vi "Write Kill Methods On Exit.vi"(8 "error in (no error)":errorcluster, 10 "Kill Methods On Exit":bool, 11 "Async Methods Actor in":refnum<class "Async Methods Actor.lvclass">) -> (0 "error out":errorcluster, 3 "Async Methods Actor out":refnum<class "Async Methods Actor.lvclass">)   [LabVIEW 2021, in "Async Methods Actor.lvlib" / "Async Methods Actor.lvclass"]
uses:
  Async Methods Actor.lvclass
  Async Methods Actor.lvclass/Async Methods Actor.ctl
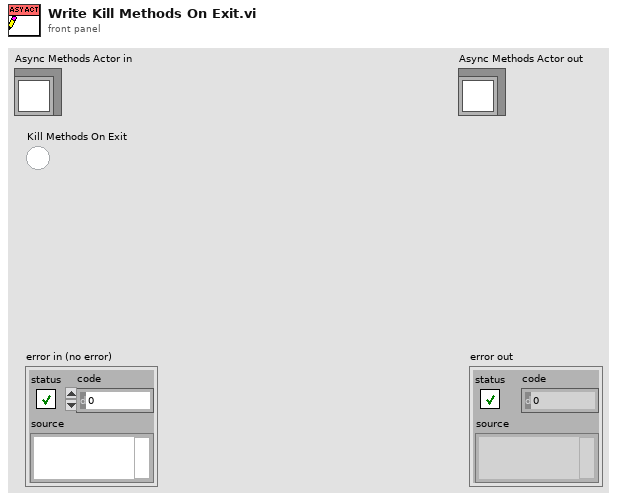
[diagram p1: front panel]
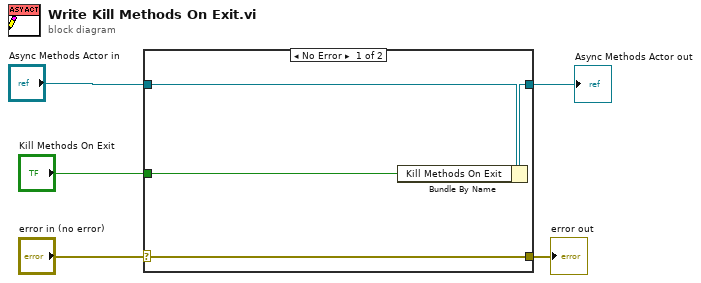
[diagram p0: block diagram]
diagram:
  n1 = case shown="No Error" "error in (no error)" {
    selector: "error in (no error)" -> [w9 w10]
    tunnel: [w9 w10] -> w4
    tunnel: [w7 w11] -> w1
    tunnel: "Async Methods Actor in" -> [w8 w11]
    tunnel: "Kill Methods On Exit" -> [w6 _]
    frame No Error {
      n2 = Bundle By Name(cluster=w8, "Kill Methods On Exit"=w6) -> (w7:refnum<class "Async Methods Actor.lvclass">)
    }
    frame Error {
    }
  }
  "error out" <- w4
  "Async Methods Actor out" <- w1
